vi "initEncoder.vi"(1 "Minimum Rate":dbl=1.0, 2 "Number Samples to Average":u8=5 min=1 max=128, 3 "refnum name":string="My Encoder RefNum", 5 "Invert Direction (False)":bool, 7 "DIO A":T2, 9 "DIO B":T2, 11 "error in (no error)":errorcluster, 12 "Circumference":dbl=12.66, 13 "Diameter (Do Not Use)":dbl, 14 "CPR":dbl=250.0) -> (15 "error out":errorcluster)   [LabVIEW 2013]
uses:
  <vilib>/Rock Robotics/SystemInterfaces/DIO/FPGA_DIOChannel.ctl
  <vilib>/Rock Robotics/WPI/Encoder/WPI_EncoderType.ctl
  <vilib>/Rock Robotics/WPI/Counter/WPI_CounterDigitalInputToDigitalSource.vi
panel:
  in  "Decoding Type":T1=enum."4x"
  # "Use only one of these. \nDiameter should be 0 \nif Circumference is used."
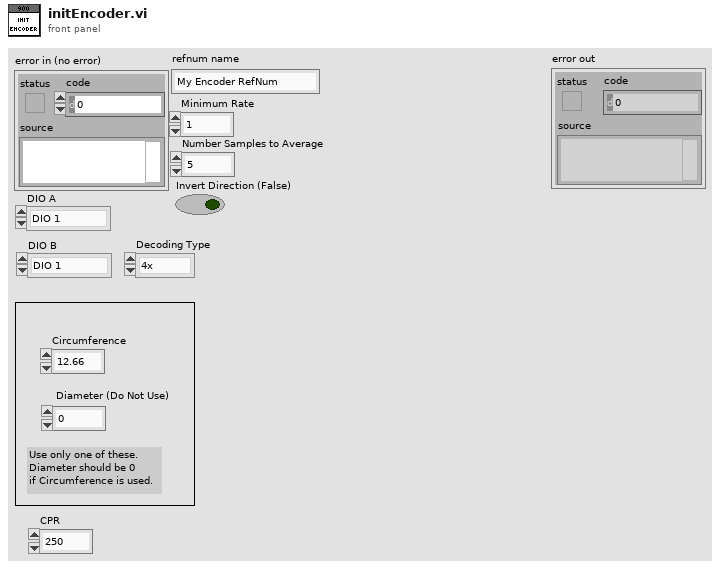
[diagram p1: front panel]
types:
  T1 = typedef "WPI_EncoderType.ctl" = enum16{"1x", "2x", "4x"}
  T2 = typedef "FPGA_DIOChannel.ctl" = enum8{"DIO 1", "DIO 2", "DIO 3", "DIO 4", "DIO 5", "DIO 6", "DIO 7", "DIO 8", "DIO 9", "DIO 10", "DIO 11", "DIO 12", "DIO 13", "DIO 14", "Invalid"}
  T3 = typedef "WPI_DigitalInputDevRef.ctl" = cluster{"DevStatus":errorcluster, "DIO Channel":T2, "Digital Module":T4}
  T4 = typedef "FPGA_TypedefDigitalModule.ctl" = enum16{"Digital Module 1", "Digital Module 2"}
  T5 = typedef "FPGA_CounterEncoderSourceConvertionLVSourceType.ctl" = cluster{"DevStatus":errorcluster, "AnalogTriggerMode?":bool, "DigitalMode":cluster{"Digital Module":T4, "DIO Channel":T6}, "AnalogTriggerMode":cluster{"AnalogTriggerIndex":T7, "OutputType":T8}}
  T6 = typedef "FPGA_DIODigitalSourceChannel.ctl" = enum8{"DIO 1", "DIO 2", "DIO 3", "DIO 4", "DIO 5", "DIO 6", "DIO 7", "DIO 8", "DIO 9", "DIO 10", "DIO 11", "DIO 12", "DIO 13", "DIO 14", "Disabled"}
  T7 = typedef "FPGA_AnalogTriggerIndex.ctl" = enum8{"Trig 0", "Trig 1", "Trig 2", "Trig 3", "Trig 4", "Trig 5", "Trig 6", "Trig 7", "Invalid"}
  T8 = typedef "FPGA_AnalogTriggerOutType.ctl" = enum16{"InWindow", "TriggerState", "Rising", "Falling"}
  T9 = typedef "WPI_EncoderDevRef.ctl" = cluster{"DevStatus":errorcluster, "EncoderIndex":T10, "CounterIndex":T11, "DistancePerCount":dbl, "Decoding Type":T1}
  T10 = typedef "FPGA_EncoderIdx.ctl" = enum8{"Enc 0", "Enc 1", "Enc 2", "Enc 3", "Invalid"}
  T11 = typedef "FPGA_CounterCtrSystemIndex.ctl" = enum8{"Ctr 0", "Ctr 1", "Ctr 2", "Ctr 3", "Ctr 4", "Ctr 5", "Ctr 6", "Ctr 7", "Invalid"}
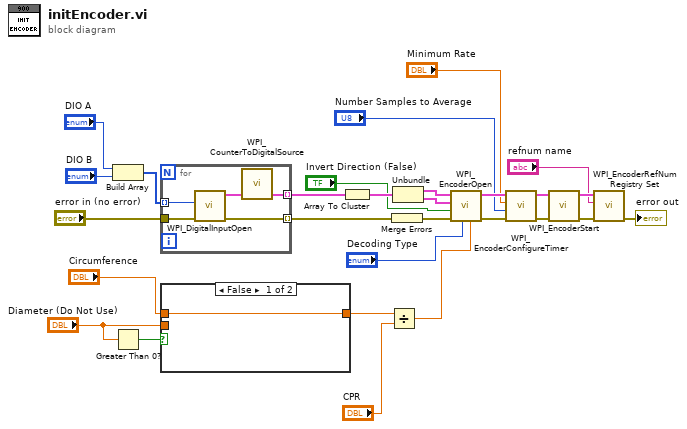
[diagram p0: block diagram]
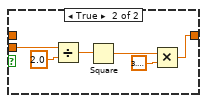
[diagram p2: hidden frame]
diagram:
  n1 = Build Array("DIO A", "DIO B") -> (w19:T2[])
  n2 = Greater Than 0?(x="Diameter (Do Not Use)") -> (x > 0?=w10:bool)
  n3 = for {
    tunnel: "error in (no error)" -> [w32]
    tunnel: w19 -> [w31] mode=indexing
    tunnel: [w30] -> w18 mode=indexing
    tunnel: [w29] -> w16 mode=indexing
    n4 = call <vilib>:"WPI_DigitalInputOpen.vi"("error in (no error)"=w32, "DIO Channel"=w31) -> ("error out"=w30:errorcluster, "DigitalInputDevRef"=w33:T3)  [unwired: 8 in]
    n5 = call-poly <vilib>:"WPI_CounterToDigitalSource.vi"("DigitalInputDevRef"=w33) -> ("Digital Source"=w29:T5)  [unwired: 6 in]
  }
  n6 = case shown="False" w10 {
    tunnel: [w34 w37] -> w8
    tunnel: "Circumference" -> [w34 _]
    tunnel: "Diameter (Do Not Use)" -> [_ w39]
    frame False {
    }
    frame True {
      n7 = Divide(x=w39, y=2.0) -> (x/y=w38:dbl)
      n8 = Square(x=w38) -> (x^2=w36:dbl)
      n9 = Multiply(x=w36, y=3.141592653589793) -> (x*y=w37:dbl)
    }
  }
  n10 = Array To Cluster(array=w16) -> (cluster=w15:cluster{"[0]":T5, "[1]":T5})
  n11 = Divide(x=w8, y="CPR") -> (x/y=w5:dbl)
  n12 = Merge Errors(w18) -> (w17:errorcluster)
  n13 = Unbundle(w15) -> ("[0]"=w14:T5, "[1]"=w13:T5)
  n14 = call <vilib>:"WPI_EncoderOpen.vi"("DistancePerCount"=w5, "Decoding Type"="Decoding Type", "error in (no error)"=w17, "Invert Direction (False)"="Invert Direction (False)", "BSource"=w13, "ASource"=w14) -> ("error out"=w26:errorcluster, "EncoderDevRef"=w25:T9)  [unwired: 4 in]
  n15 = call <vilib>:"WPI_EncoderConfigureTimer.vi"("error in (no error)"=w26, "Number Samples to Average"="Number Samples to Average", "Minimum Rate"="Minimum Rate", "EncoderDevRef"=w25) -> ("error out"=w28:errorcluster, "EncoderDevRef"=w27:T9)  [unwired: 6 in]
  n16 = call <vilib>:"WPI_EncoderStart.vi"("error in (no error)"=w28, "EncoderDevRef"=w27) -> ("error out"=w23:errorcluster, "EncoderDevRef"=w24:T9)  [unwired: 8 in]
  n17 = call <vilib>:"WPI_EncoderRefNum Registry Set.vi"("error in (no error)"=w23, "refnum name"="refnum name", "EncoderDevRef"=w24) -> ("error out"=→"error out":errorcluster)  [unwired: 7 in, 1 out]
